vi "Add Tree Level.vi"(0 "tdms file":refnum<k34>, 1 "Tree Refnum":refnum<vi>, 2 "Relative File Path":string, 3 "Property Name":string, 5 "Tree Parent Tags In":string[](array[string]), 7 "Tree Items Created In":variant, 9 "Group/Channel Names In":string[](array[string]), 11 "error in (no error)":errorcluster, 12 "Hide Undefined Channels":bool) -> (4 "tdms file out":refnum<k34>, 6 "Tree Parent Tags Out":string[](array[string]), 8 "Tree Items Created Out":variant, 10 "Group/Channel Names Out":string[](array[string]), 15 "error out":errorcluster)   [LabVIEW 2017, in "XTree.xctl"]
doc: "Creates a hierarchical \"level\" in the tree according to the specified property."
uses:
  <vilib>/addons/_NIFileIO/XTree/XTree.xctl
panel:
  # "Array of the lowest level tree locations for each channel which have been created so far"
  # "Property which this level will be based upon"
  # "An array of tree locations which have been created. Used to prevent duplicate tree locations."
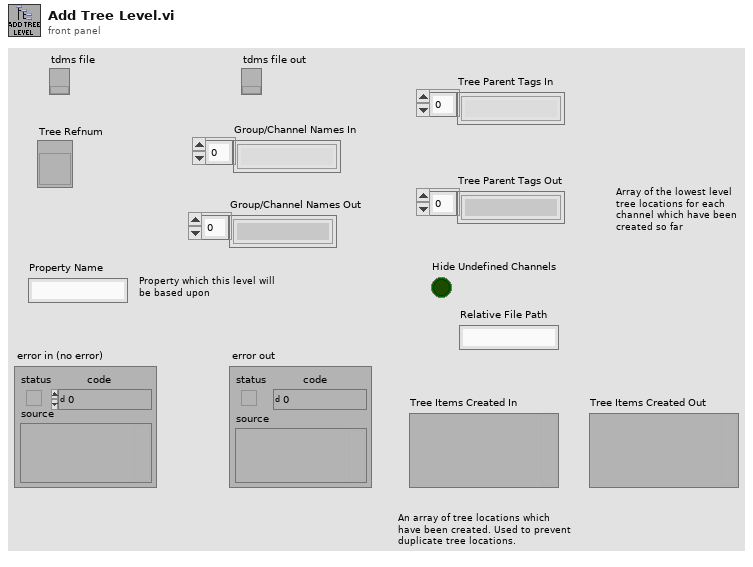
[diagram p1: front panel]
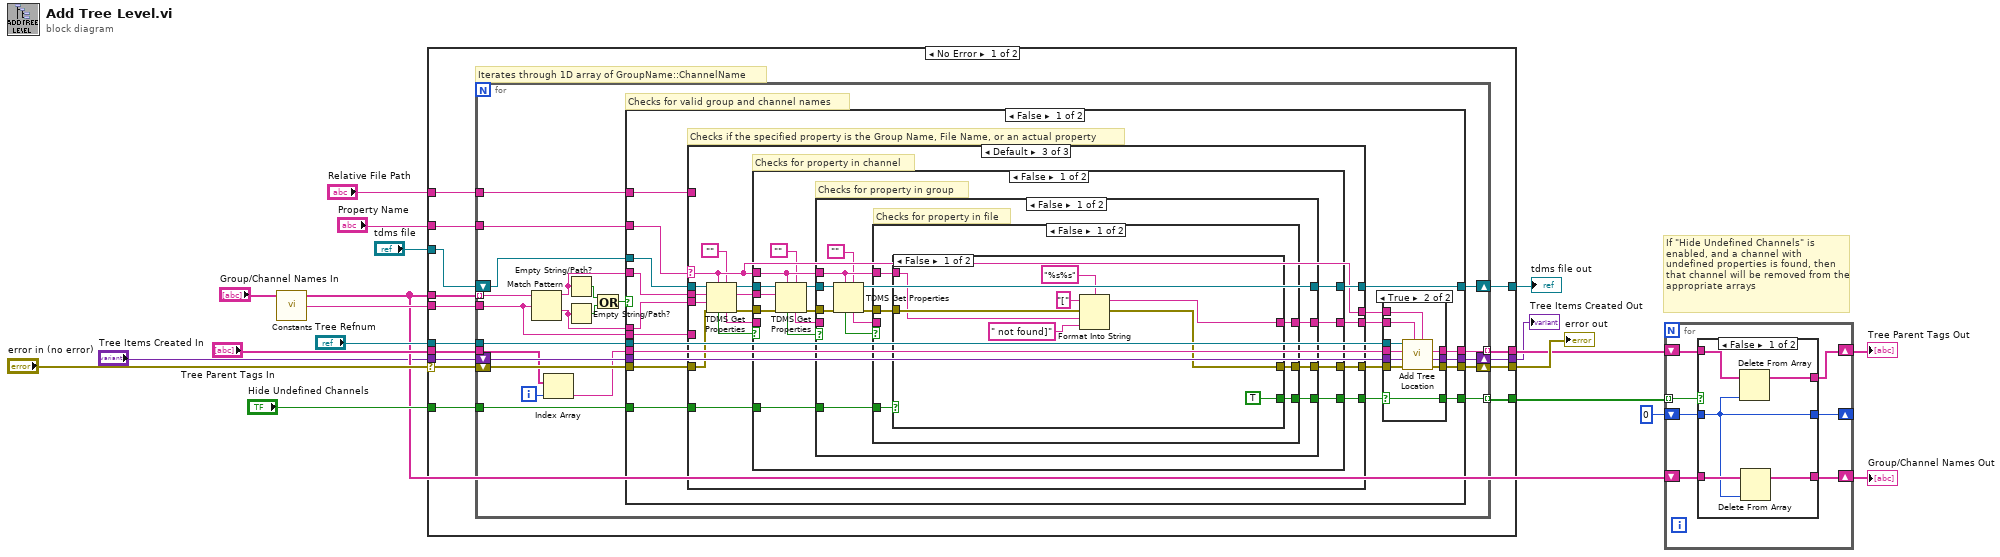
[diagram p0: block diagram]
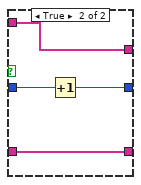
[diagram p2: hidden frame]
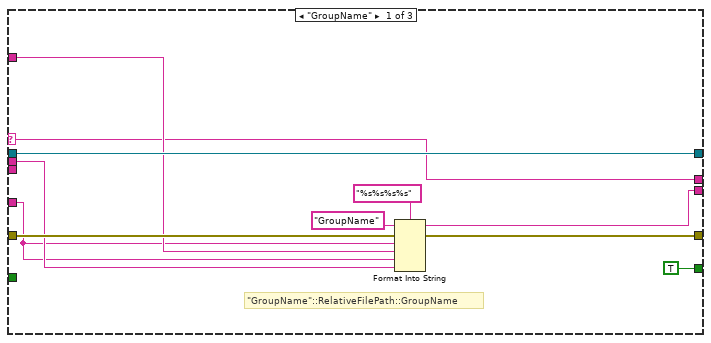
[diagram p4: hidden frame]
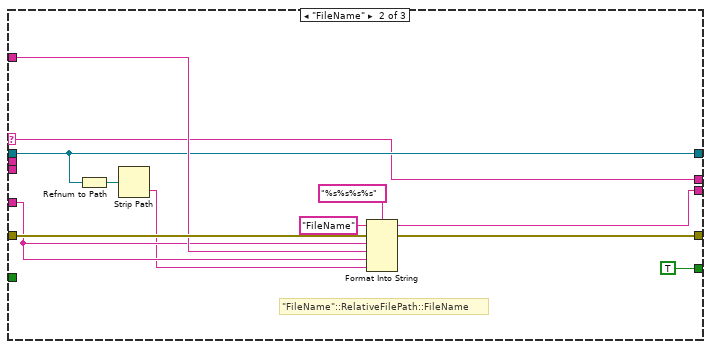
[diagram p5: hidden frame]
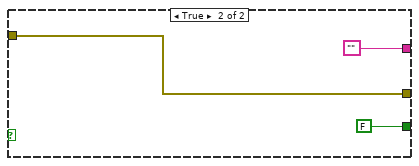
[diagram p6: hidden frame]
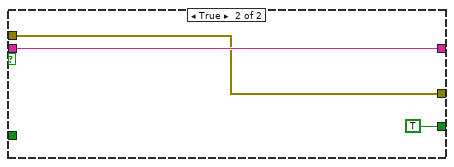
[diagram p7: hidden frame]
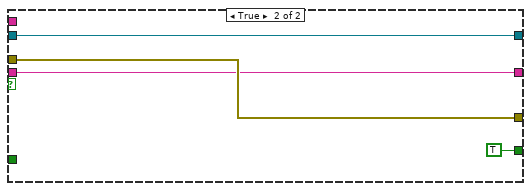
[diagram p8: hidden frame]
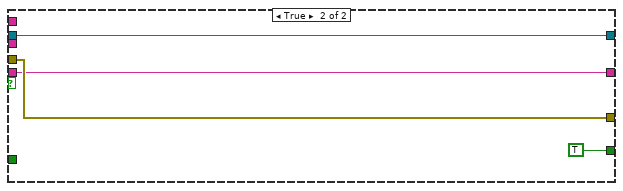
[diagram p9: hidden frame]
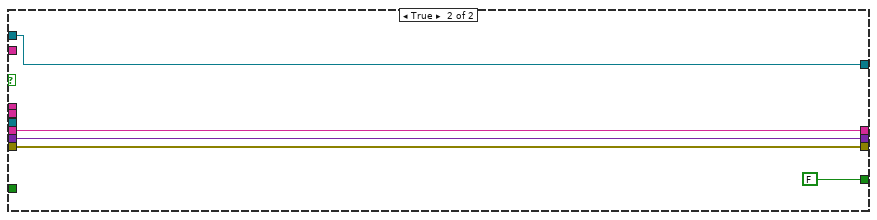
[diagram p10: hidden frame]
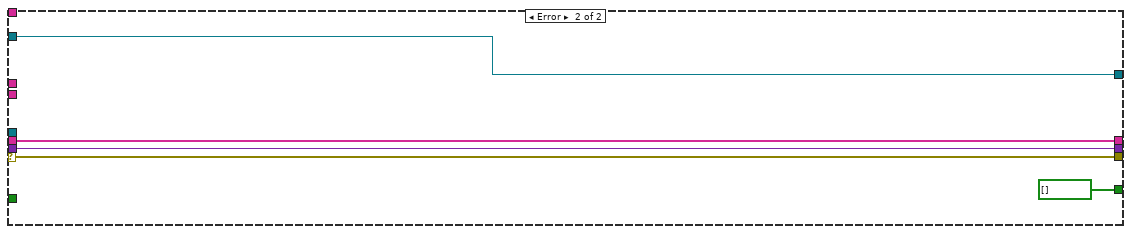
[diagram p11: hidden frame]
diagram:
  # "If \"Hide Undefined Channels\" is enabled, and a channel with undefined properties is found, then that channel will be removed from the appropriate arrays"
  n1 = call <vilib>:"Constants.vi"() -> ("String Delimeter"=w13:string)  [unwired: 5 in]
  n2 = case shown="No Error" "error in (no error)" {
    selector: "error in (no error)" -> [w24 w189]
    tunnel: "Tree Refnum" -> [w33 _]
    tunnel: "Tree Parent Tags In" -> [w32 w191]
    tunnel: "Tree Items Created In" -> [w31 w190]
    tunnel: "tdms file" -> [w30 w192]
    tunnel: [w29 w189] -> w15
    tunnel: [w28 w190] -> w1
    tunnel: [w27 w191] -> w8
    tunnel: [w26 w192] -> w14
    tunnel: w13 -> [w25 _]
    tunnel: "Group/Channel Names In" -> [w23 _]
    tunnel: "Property Name" -> [w22 _]
    tunnel: "Hide Undefined Channels" -> [w21 _]
    tunnel: [w20 bool[] []] -> w9
    tunnel: "Relative File Path" -> [w19 _]
    frame No Error {
      # "Iterates through 1D array of GroupName::ChannelName"
      n3 = for {
        tunnel: w23 -> [w37] mode=indexing
        tunnel: w22 -> [w50]
        tunnel: w33 -> [w49]
        tunnel: w32 -> [w40]
        shift-right: [w46] -> w26
        shift-left: w30 -> [w47]
        shift-right: [w44] -> w29
        shift-left: w24 -> [w45]
        shift-right: [w43] -> w28
        shift-left: w31 -> [w48]
        tunnel: [w42] -> w27 mode=indexing
        tunnel: w25 -> [w35]
        tunnel: w21 -> [w38]
        tunnel: [w36] -> w20 mode=indexing
        tunnel: w19 -> [w34]
        i -> [w41]
        # "Checks for valid group and channel names"
        n4 = Match Pattern(string=w37, regular expression=w35) -> (before substring=w52:string, after substring=w51:string)  [unwired: 1 in, 2 out]
        n5 = Index Array(array=w40, index=w41) -> (element=w39:string)
        n6 = Empty String/Path?(string/path=w52) -> (empty?=w54:bool)
        n7 = Empty String/Path?(string/path=w51) -> (empty?=w53:bool)
        n8 = Or(x=w54, y=w53) -> (x .or. y?=w55:bool)
        n9 = case shown="False" w55 {
          tunnel: w52 -> [w75 _]
          tunnel: w51 -> [w74 _]
          tunnel: w50 -> [w73 _]
          tunnel: w49 -> [w60 _]
          tunnel: w39 -> [w61 w185]
          tunnel: w48 -> [w62 w186]
          tunnel: w47 -> [w72 w184]
          tunnel: [w59 w184] -> w46
          tunnel: w45 -> [w71 w187]
          tunnel: [w68 w187] -> w44
          tunnel: [w67 w186] -> w43
          tunnel: [w66 w185] -> w42
          tunnel: w38 -> [w65 _]
          tunnel: [w63 FALSE] -> w36
          tunnel: w35 -> [w58 _]
          tunnel: w34 -> [w57 _]
          frame False {
            # "Checks if the specified property is the Group Name, File Name, or an actual property"
            n10 = case shown="Default" w73 {
              selector: w73 -> [w90 w101 w114]
              tunnel: w75 -> [w94 _ w126]
              tunnel: w74 -> [_ _ w125]
              tunnel: w72 -> [w100 w107 w122]
              tunnel: [w100 w107 w121] -> w59
              tunnel: w71 -> [w98 w111 w119]
              tunnel: [w97 w110 w118] -> w69
              tunnel: [w93 w103 w117] -> w70
              tunnel: w65 -> [_ _ w116]
              tunnel: [TRUE TRUE w115] -> w64
              tunnel: w58 -> [w91 w105 _]
              tunnel: w57 -> [w95 w108 _]
              tunnel: [w90 w101 w114] -> w56
              frame "GroupName" {
                # "\"GroupName\"::RelativeFilePath::GroupName"
                n11 = Format Into String(format string="%s%s%s%s", initial string="GroupName", error in=w98, w91, w95, w91, w94) -> (resulting string=w93:string, error out=w97:errorcluster)
              }
              frame "FileName" {
                # "\"FileName\"::RelativeFilePath::FileName"
                n12 = Refnum to Path(1:w107) -> (0:w106:path)
                n13 = Strip Path(path=w106) -> (name=w104:string)  [unwired: 1 out]
                n14 = Format Into String(format string="%s%s%s%s", initial string="FileName", error in=w111, w105, w108, w105, w104) -> (resulting string=w103:string, error out=w110:errorcluster)
              }
              frame Default {
                # "Checks for property in channel"
                n15 = TDMS Get Properties(5:"", 7:w114, 8:w119, 9:w125, 10:w126, 11:w122) -> (0:w128:errorcluster, 2:w127:string, 3:w124:refnum<k34>, 4:w120:string, 6:w123:bool)  [unwired: 1 out]
                n16 = case shown="False" w123 {
                  tunnel: w128 -> [w142 w181]
                  tunnel: w114 -> [w137 _]
                  tunnel: [w136 w182] -> w121
                  tunnel: [w135 w181] -> w118
                  tunnel: w127 -> [w134 _]
                  tunnel: w124 -> [w133 w182]
                  tunnel: w120 -> [_ w180]
                  tunnel: [w132 w180] -> w117
                  tunnel: w116 -> [w131 _]
                  tunnel: [w130 TRUE] -> w115
                  frame False {
                    # "Checks for property in group"
                    n17 = TDMS Get Properties(5:"", 7:w137, 8:w142, 10:w134, 11:w133) -> (0:w139:errorcluster, 3:w138:refnum<k34>, 4:w140:string, 6:w141:bool)  [unwired: 1 in, 2 out]
                    n18 = case shown="False" w141 {
                      tunnel: w140 -> [_ w177]
                      tunnel: w139 -> [w153 w178]
                      tunnel: w138 -> [w154 w175]
                      tunnel: w137 -> [w145 _]
                      tunnel: [w149 w178] -> w135
                      tunnel: [w144 w175] -> w136
                      tunnel: [w148 w177] -> w132
                      tunnel: w131 -> [w147 _]
                      tunnel: [w146 TRUE] -> w130
                      frame False {
                        # "Checks for property in file"
                        n19 = TDMS Get Properties(5:"", 7:w145, 8:w153, 11:w154) -> (0:w151:errorcluster, 3:w144:refnum<k34>, 4:w150:string, 6:w152:bool)  [unwired: 2 in, 2 out]
                        n20 = case shown="False" w152 {
                          tunnel: w151 -> [w157 w173]
                          tunnel: w150 -> [_ w174]
                          tunnel: [w158 w173] -> w149
                          tunnel: [w160 w174] -> w148
                          tunnel: w147 -> [w159 _]
                          tunnel: [w156 TRUE] -> w146
                          tunnel: w145 -> [w155 _]
                          frame False {
                            n21 = case shown="False" w159 {
                              tunnel: [w167 ""] -> w160
                              tunnel: [w165 w170] -> w158
                              tunnel: w157 -> [w166 w170]
                              tunnel: [TRUE FALSE] -> w156
                              tunnel: w155 -> [w161 _]
                              frame False {
                                n22 = Format Into String(format string="%s%s", initial string="[", error in=w166, w161, " not found]" ("input 2")) -> (resulting string=w167:string, error out=w165:errorcluster)
                              }
                              frame True {
                              }
                            }
                          }
                          frame True {
                          }
                        }
                      }
                      frame True {
                      }
                    }
                  }
                  frame True {
                  }
                }
              }
            }
            n23 = case shown="True" w64 {
              selector: w64 -> [w76 w81]
              tunnel: w70 -> [_ w89]
              tunnel: w60 -> [_ w88]
              tunnel: w61 -> [w79 w87]
              tunnel: w62 -> [w78 w86]
              tunnel: w69 -> [w77 w85]
              tunnel: [w77 w84] -> w68
              tunnel: [w78 w83] -> w67
              tunnel: [w79 w82] -> w66
              tunnel: [w76 w81] -> w63
              tunnel: w56 -> [_ w80]
              frame False {
              }
              frame True {
                n24 = call <vilib>:"Add Tree Location.vi"("Property Name"=w80, "Property Value"=w89, "error in (no error)"=w85, "Tree Items Created In"=w86, "Tree Parent Tag In"=w87, "TreeControl in"=w88) -> ("error out"=w84:errorcluster, "Tree Items Created Out"=w83:variant, "Tree Parent Tag Out"=w82:string)  [unwired: 3 in]
              }
            }
          }
          frame True {
          }
        }
      }
    }
    frame Error {
    }
  }
  "error out" <- w15
  "tdms file out" <- w14
  "Tree Items Created Out" <- w1
  n25 = for {
    tunnel: w9 -> [w199] mode=indexing
    shift-right: [w197] -> w7
    shift-left: w8 -> [w198]
    shift-right: [w195] -> _
    shift-left: 0 -> [w196]
    shift-right: [w193] -> w4
    shift-left: "Group/Channel Names In" -> [w194]
    n26 = case shown="False" w199 {
      tunnel: w198 -> [w204 w208]
      tunnel: [w203 w208] -> w197
      tunnel: w196 -> [w201 w207]
      tunnel: [w201 w206] -> w195
      tunnel: w194 -> [w202 w205]
      tunnel: [w200 w205] -> w193
      frame False {
        n27 = Delete From Array(array=w204, index=w201) -> (array with subset deleted=w203:string[])  [unwired: 1 in, 1 out]
        n28 = Delete From Array(array=w202, index=w201) -> (array with subset deleted=w200:string[])  [unwired: 1 in, 1 out]
      }
      frame True {
        n29 = Increment(x=w207) -> (x+1=w206:i32)
      }
    }
  }
  "Tree Parent Tags Out" <- w7
  "Group/Channel Names Out" <- w4
